vi "Single_Omit.vi"(3 "Accept In":bool[](array[boolean]), 4 "Data Values":string[](array[string]), 5 "Omit Strings":string[](array[string])) -> (0 "Accept Out":bool[](array[boolean]))   [LabVIEW 2010]
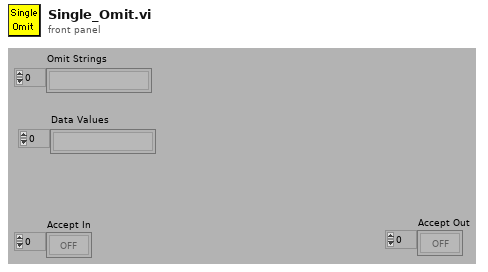
[diagram p1: front panel]
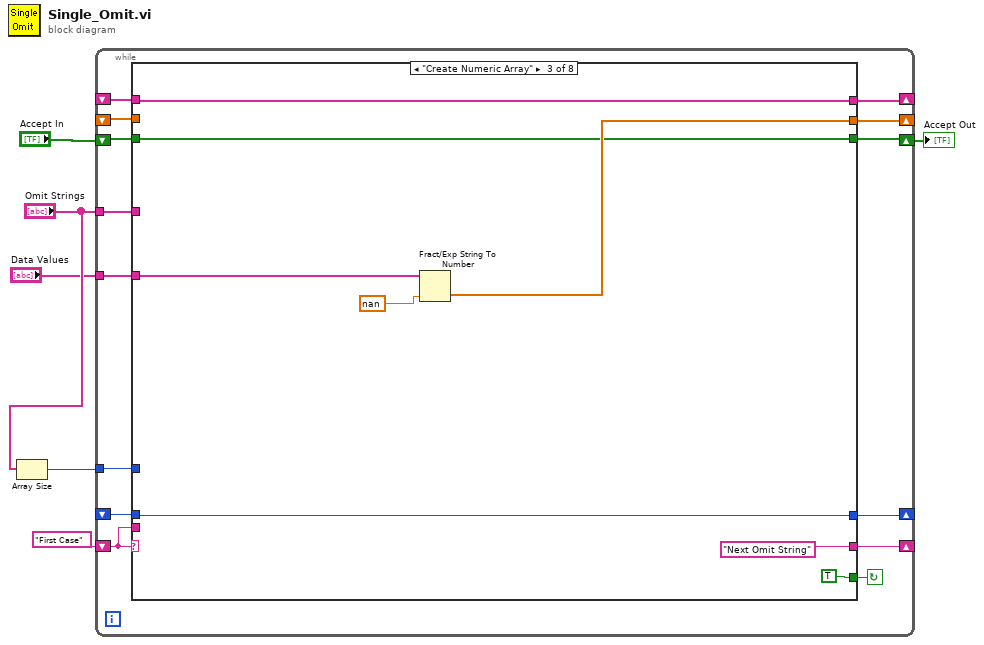
[diagram p0: block diagram]
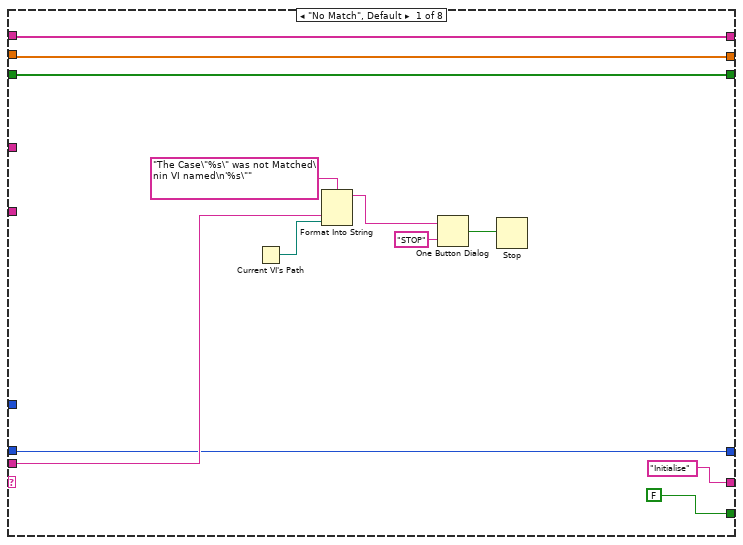
[diagram p2: hidden frame]
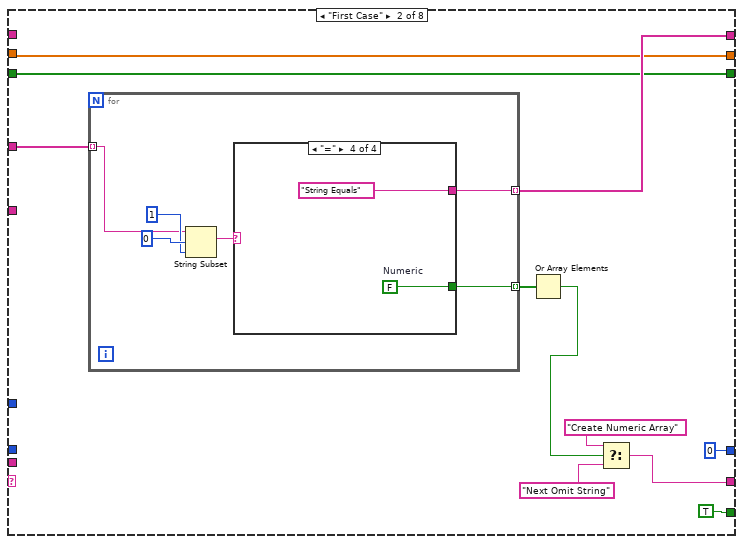
[diagram p3: hidden frame]
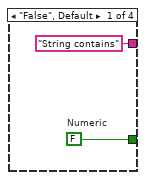
[diagram p4: hidden frame]
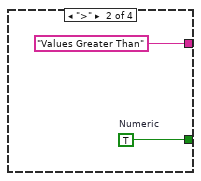
[diagram p5: hidden frame]
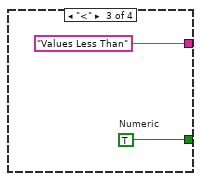
[diagram p6: hidden frame]
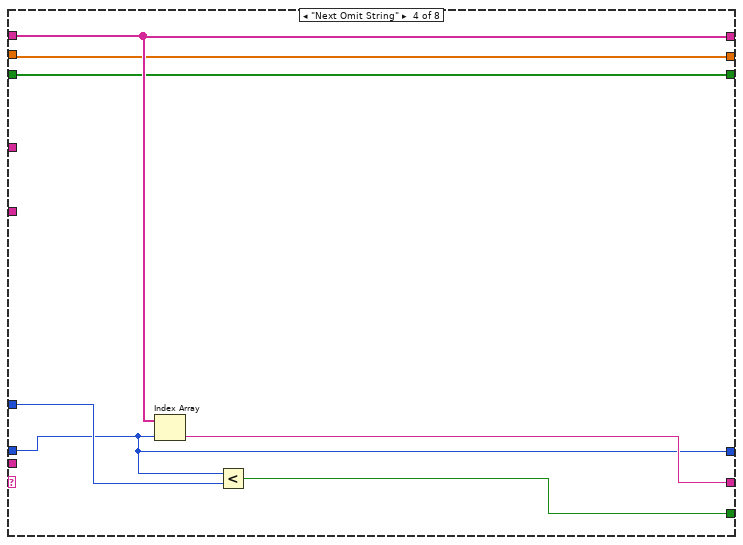
[diagram p7: hidden frame]
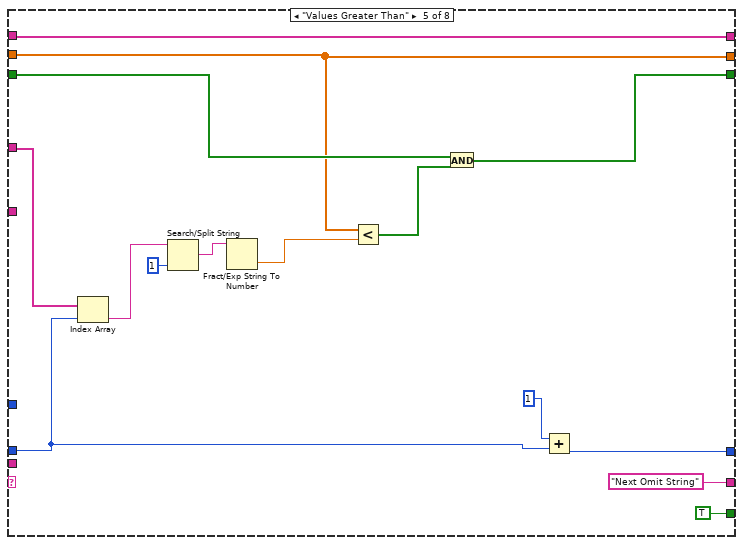
[diagram p8: hidden frame]
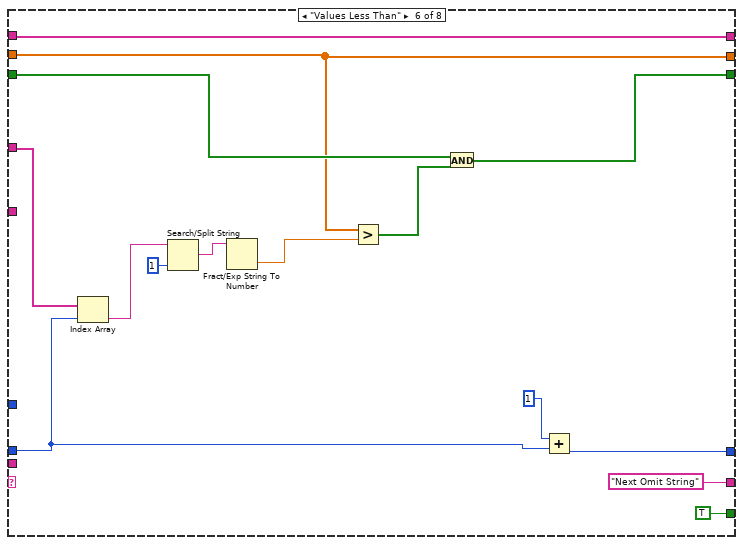
[diagram p9: hidden frame]
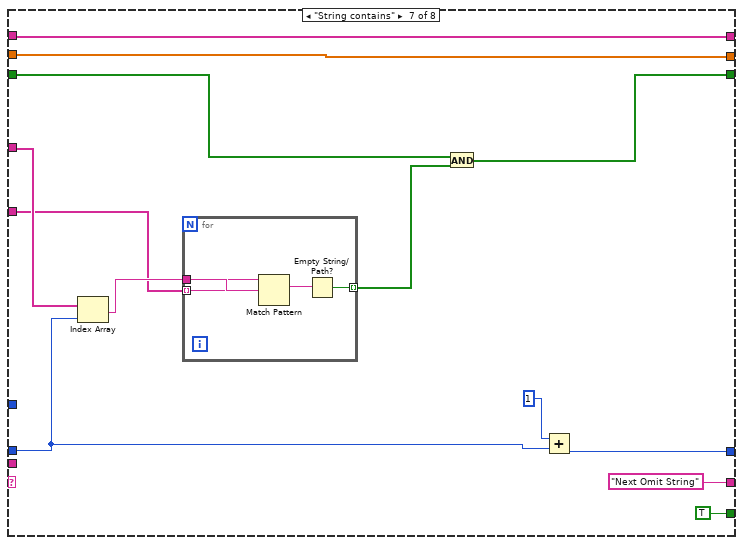
[diagram p10: hidden frame]
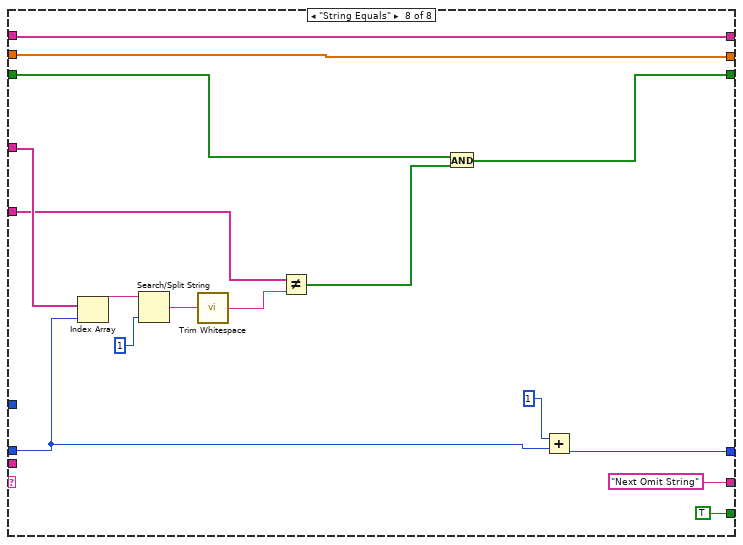
[diagram p11: hidden frame]
diagram:
  n1 = Array Size(array="Omit Strings") -> (size(s)=w3:i32)
  n2 = while {
    shift-left: "Accept In" -> [w7]
    shift-right: [w8] -> w2
    tunnel: w3 -> [w10]
    shift-left: _ -> [w9]
    shift-right: [w11] -> _
    tunnel: "Data Values" -> [w12]
    shift-left: _ -> [w13]
    shift-right: [w14] -> _
    tunnel: "Omit Strings" -> [w15]
    shift-left: _ -> [w17]
    shift-right: [w16] -> _
    shift-left: "First Case" -> [w18]
    shift-right: [w19] -> _
    stop <- w20 continue-if-true
    n3 = case shown="\"Create Numeric Array\"" w18 {
      tunnel: [FALSE TRUE TRUE w71 TRUE TRUE TRUE TRUE] -> w20
      tunnel: ["Initialise" w36 "Next Omit String" w70 "Next Omit String" "Next Omit String" "Next Omit String" "Next Omit String"] -> w19
      tunnel: w18 -> [w27 _ _ _ _ _ _ _]
      tunnel: w17 -> [w24 _ w60 w68 w78 w93 w112 w132]
      tunnel: [w24 w37 w60 w68 w78 w93 w112 w132] -> w16
      tunnel: w15 -> [_ w42 _ _ w86 w101 w115 w135]
      tunnel: [w21 0 w62 w69 w75 w90 w109 w129] -> w14
      tunnel: w13 -> [w21 _ w62 w69 w77 w92 w111 w131]
      tunnel: w12 -> [_ _ w64 _ _ _ w104 w121]
      tunnel: [w23 w35 w63 w67 w79 w94 w106 w126] -> w11
      tunnel: w10 -> [_ _ _ w72 _ _ _ _]
      tunnel: w9 -> [w23 w35 _ w67 w79 w94 w106 w126]
      tunnel: [w22 w33 w59 w66 w80 w95 w113 w133] -> w8
      tunnel: w7 -> [w22 w33 w59 w66 w81 w96 w114 w134]
      frame "No Match", Default {
        n4 = Current VI's Path() -> (path=w26:path)
        n5 = Format Into String(format string="The Case\"%s\" was not Matched\nin VI named\n'%s\"" ("Format String"), w27, w26) -> (resulting string=w30:string)  [unwired: 2 in, 1 out]
        n6 = One Button Dialog(message=w30, button name ("OK")="STOP") -> (true=w28:bool)
        n7 = Stop(stop? (T)=w28) -> ()
      }
      frame "First Case" {
        n8 = for {
          tunnel: w42 -> [w46] mode=indexing
          tunnel: [w45] -> w37 mode=indexing
          tunnel: [w44] -> w41 mode=indexing
          n9 = String Subset(string=w46, offset (0)=0, length (rest)=1 ("length")) -> (substring=w47:string)
          n10 = case shown="\"=\"" w47 {
            tunnel: ["String contains" "Values Greater Than" "Values Less Than" "String Equals"] -> w45
            tunnel: [w50 w52 w54 w56] -> w44
            frame "False", Default {
              w50 = FALSE  # Numeric
            }
            frame ">" {
              w52 = TRUE  # Numeric
            }
            frame "<" {
              w54 = TRUE  # Numeric
            }
            frame "=" {
              w56 = FALSE  # Numeric
            }
          }
        }
        n11 = Or Array Elements(Boolean array=w41) -> (logical OR=w40:bool)
        n12 = Select(t="Create Numeric Array", s=w40, f="Next Omit String") -> (s? t:f=w36:string)
      }
      frame "Create Numeric Array" {
        n13 = Fract/Exp String To Number(string=w64, default (0 dbl)=nan) -> (number=w63:dbl[])  [unwired: 3 out]
      }
      frame "Next Omit String" {
        n14 = Index Array(array=w68, index=w69) -> (element=w70:string)
        n15 = Less?(x=w69, y=w72) -> (x < y?=w71:bool)
      }
      frame "Values Greater Than" {
        n16 = Index Array(array=w86, index=w77) -> (element=w85:string)
        n17 = Search/Split String(string=w85, offset (0)=1) -> (match + rest of string=w84:string)  [unwired: 3 out]
        n18 = Fract/Exp String To Number(string=w84) -> (number=w83:dbl)  [unwired: 4 out]
        n19 = Less?(x=w79, y=w83) -> (x < y?=w82:bool[])
        n20 = And(x=w81, y=w82) -> (x .and. y?=w80:bool[])
        n21 = Add(x=1, y=w77) -> (x+y=w75:i32)
      }
      frame "Values Less Than" {
        n22 = Index Array(array=w101, index=w92) -> (element=w100:string)
        n23 = Search/Split String(string=w100, offset (0)=1) -> (match + rest of string=w99:string)  [unwired: 3 out]
        n24 = Fract/Exp String To Number(string=w99) -> (number=w98:dbl)  [unwired: 4 out]
        n25 = Greater?(x=w94, y=w98) -> (0:w97:bool[])
        n26 = And(x=w96, y=w97) -> (x .and. y?=w95:bool[])
        n27 = Add(x=1, y=w92) -> (x+y=w90:i32)
      }
      frame "String contains" {
        n28 = Index Array(array=w115, index=w111) -> (element=w105:string)
        n29 = for {
          tunnel: w105 -> [w119]
          tunnel: w104 -> [w118] mode=indexing
          tunnel: [w116] -> w103 mode=indexing
          n30 = Match Pattern(string=w118, regular expression=w119) -> (match substring=w117:string)  [unwired: 4 out]
          n31 = Empty String/Path?(string/path=w117) -> (empty?=w116:bool)
        }
        n32 = And(x=w114, y=w103) -> (x .and. y?=w113:bool[])
        n33 = Add(x=1, y=w111) -> (x+y=w109:i32)
      }
      frame "String Equals" {
        n34 = Index Array(array=w135, index=w131) -> (element=w124:string)
        n35 = Search/Split String(string=w124, offset (0)=1) -> (match + rest of string=w123:string)  [unwired: 3 out]
        n36 = call <vilib>:"Trim Whitespace.vi"("string"=w123) -> ("trimmed string"=w122:string)  [unwired: 1 in]
        n37 = Not Equal?(x=w121, y=w122) -> (x != y?=w120:bool[])
        n38 = And(x=w134, y=w120) -> (x .and. y?=w133:bool[])
        n39 = Add(x=1, y=w131) -> (x+y=w129:i32)
      }
    }
  }
  "Accept Out" <- w2
